vi "Classes Initialization.vi"(7 "LabVIEW Icon in":string, 8 "error in (no error)":errorcluster {"code" min=0 max=0}, 10 "User events":T8, 11 "Ref Cluster":T3) -> (0 "error out":errorcluster {"code" min=0 max=0}, 3 "Data out":T1={"Class"={"Ants"=refnum, "Layer"=refnum, "Templates"=refnum, "Icon"=refnum, "Glyph"=refnum, "Settings"=refnum, "Tools"=refnum}, "Ref"={"Add Layer"=refnum, "Remove Layer"=refnum, "Line Text"=[], "Body Text Spec"=refnum, "DNL_Font"=refnum, "glyph path str"=refnum, "templates path str"=refnum, "Arrow Up"=refnum, "Arrow Down"=refnum, "IE VI Ref"=refnum, "Glyphs tree"=refnum, "Templates tree"=refnum, "Layer Icon Text"=refnum, "Layer Template"=refnum, "Clipboard"=refnum, "BW icon in"=refnum, "Color icon in"=refnum, "Layer Clust"=refnum, "Body Text"=refnum, "DNL_Framework Templates"=refnum, "Search Templates"=refnum, "TextMarker"=refnum, "Tab Control"=refnum, "Search Glyphs"=refnum, "Line Color"=refnum, "DNL_Glyphs []"=refnum, "Fill Color"=refnum, "Tools"=refnum, "Glyphs tree"=refnum, "Icon"=refnum, "Preview"=refnum, "Ants"=refnum, "Terminals"=refnum, "menu reference"=refnum, "LayerNames"=[], "GlyphLoadAnimation"=refnum, "TemplateLoadAnimation"=refnum, "refreshGlyphs"=refnum, "refreshTemplates"=refnum}, "Support"={"AntsRect"={"left"=0, "top"=0, "right"=0, "bottom"=0}, "Mouse Move Coords"={"Horizontal"=0, "Vertical"=0}, "Mouse Down Coords"={"Horizontal"=0, "Vertical"=0}, "Temp Coord"={"Horizontal"=0, "Vertical"=0}, "Action"=enum."Default", "Edge Color"=4914962, "Fill Color"=16860, "Mouse Down?"=FALSE, "Draft Mode?"=FALSE, "Temp Icon"=bytes[3102], "CTRL Pressed"=FALSE, "Move Selection?"=FALSE, "AntsRect Orig"={"left"=0, "top"=0, "right"=0, "bottom"=0}, "Text"="", "TM Set?"=FALSE, "Mouse inside icon?"=FALSE, "Tool (old value)"=0, "Pencil Move Color"=0, "Swap Colors?"=FALSE, "Shift pressed?"=FALSE}})   [LabVIEW 2021]
uses:
  <resource>/plugins/NIIconEditor/Controls/References Cluster.ctl
  <resource>/plugins/NIIconEditor/Controls/IE Data.ctl
  <resource>/plugins/NIIconEditor/Class/Ants/Ants.lvclass
  <resource>/plugins/NIIconEditor/Class/FakedArray/FakedArray.lvclass
  <resource>/plugins/NIIconEditor/Class/Icon Library/Glyph.lvclass
  <resource>/plugins/NIIconEditor/Class/Settings/Settings.lvclass
  <resource>/plugins/NIIconEditor/Class/Tools/Tools Paint.lvclass
  <vilib>/LabVIEW Icon API/lv_icon/Classes/Icon/Icon.lvclass
  <resource>/plugins/NIIconEditor/Controls/IE Classes.ctl
  <resource>/plugins/NIIconEditor/Controls/SupportClass.ctl
  <vilib>/Utility/miscctls.llb/LVPoint32TypeDef.ctl
  <resource>/plugins/NIIconEditor/Controls/SupportClass_Action.ctl
  <vilib>/LabVIEW Icon API/lv_icon/Controls/IEColor.ctl
  <resource>/plugins/NIIconEditor/Controls/ToMoreSpecific_Faked2DArray.ctl
  <resource>/plugins/NIIconEditor/Controls/Undo Redo Action.ctl
  <resource>/plugins/NIIconEditor/Global Variables/Data.vi
panel:
  in  "Data":T1={"Class"={"Ants"=refnum, "Layer"=refnum, "Templates"=refnum, "Icon"=refnum, "Glyph"=refnum, "Settings"=refnum, "Tools"=refnum}, "Ref"={"Add Layer"=refnum, "Remove Layer"=refnum, "Line Text"=[], "Body Text Spec"=refnum, "DNL_Font"=refnum, "glyph path str"=refnum, "templates path str"=refnum, "Arrow Up"=refnum, "Arrow Down"=refnum, "IE VI Ref"=refnum, "Glyphs tree"=refnum, "Templates tree"=refnum, "Layer Icon Text"=refnum, "Layer Template"=refnum, "Clipboard"=refnum, "BW icon in"=refnum, "Color icon in"=refnum, "Layer Clust"=refnum, "Body Text"=refnum, "DNL_Framework Templates"=refnum, "Search Templates"=refnum, "TextMarker"=refnum, "Tab Control"=refnum, "Search Glyphs"=refnum, "Line Color"=refnum, "DNL_Glyphs []"=refnum, "Fill Color"=refnum, "Tools"=refnum, "Glyphs tree"=refnum, "Icon"=refnum, "Preview"=refnum, "Ants"=refnum, "Terminals"=refnum, "menu reference"=refnum, "LayerNames"=[], "GlyphLoadAnimation"=refnum, "TemplateLoadAnimation"=refnum, "refreshGlyphs"=refnum, "refreshTemplates"=refnum}, "Support"={"AntsRect"={"left"=0, "top"=0, "right"=0, "bottom"=0}, "Mouse Move Coords"={"Horizontal"=0, "Vertical"=0}, "Mouse Down Coords"={"Horizontal"=0, "Vertical"=0}, "Temp Coord"={"Horizontal"=0, "Vertical"=0}, "Action"=enum."Default", "Edge Color"=4914962, "Fill Color"=16860, "Mouse Down?"=FALSE, "Draft Mode?"=FALSE, "Temp Icon"=bytes[3102], "CTRL Pressed"=FALSE, "Move Selection?"=FALSE, "AntsRect Orig"={"left"=0, "top"=0, "right"=0, "bottom"=0}, "Text"="", "TM Set?"=FALSE, "Mouse inside icon?"=FALSE, "Tool (old value)"=0, "Pencil Move Color"=0, "Swap Colors?"=FALSE, "Shift pressed?"=FALSE}}
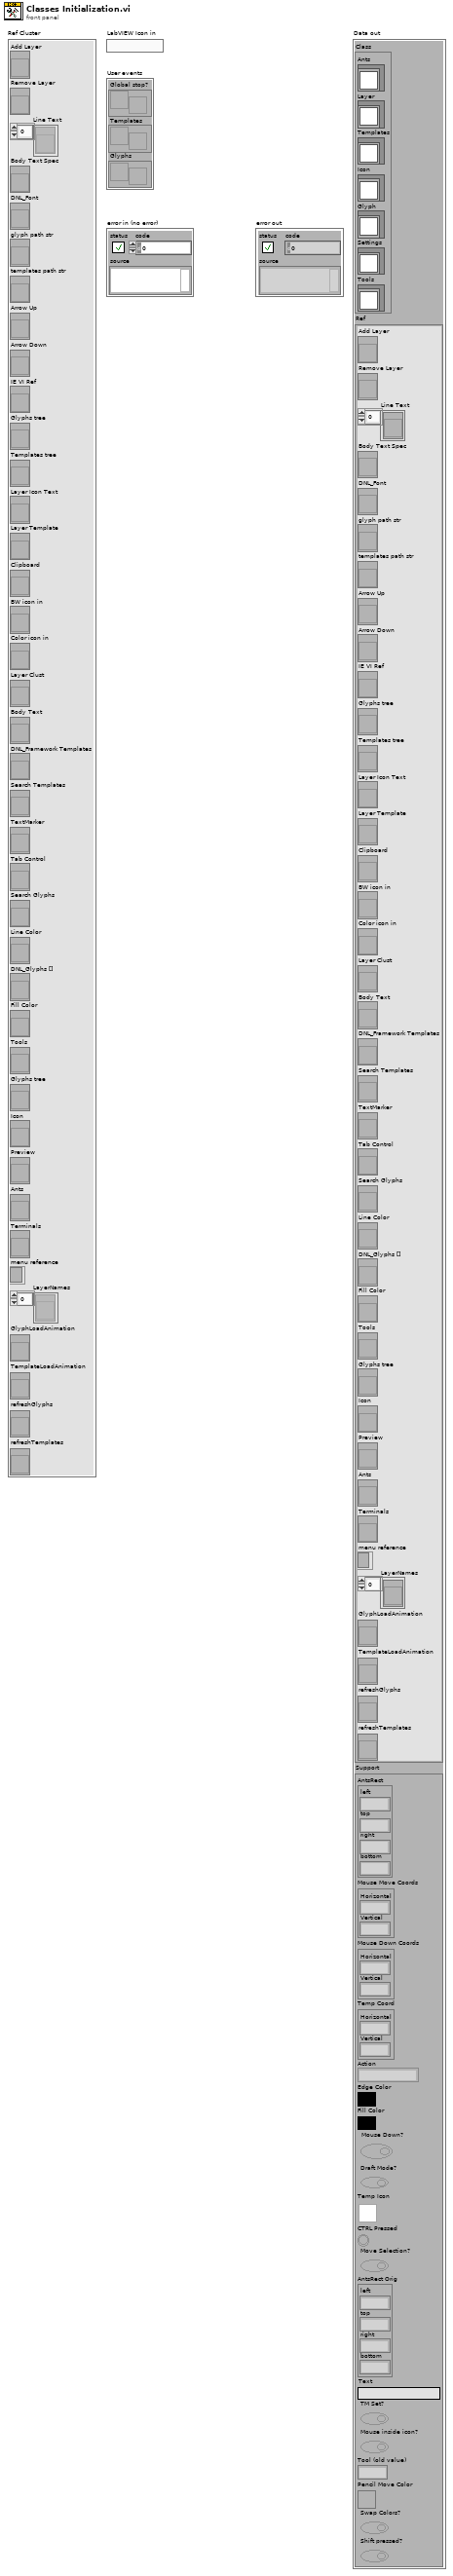
[diagram p1: front panel]
types:
  T1 = typedef "IE Data.ctl" = cluster{"Class":T2, "Ref":T3, "Support":T4}
  T2 = typedef "IE Classes.ctl" = cluster{"Ants":refnum<class "Ants.lvclass">, "Layer":refnum<class "FakedArray.lvclass">, "Templates":refnum<class "FakedArray.lvclass">, "Icon":refnum<class "Icon.lvclass">, "Glyph":refnum<class "Glyph.lvclass">, "Settings":refnum<class "Settings.lvclass">, "Tools":refnum<class "Tools Paint.lvclass">}
  T3 = typedef "References Cluster.ctl" = cluster{"Add Layer":refnum<vi>, "Remove Layer":refnum<vi>, "Line Text":refnum<vi>[], "Body Text Spec":refnum<vi>, "DNL_Font":refnum<vi>, "glyph path str":refnum<vi>, "templates path str":refnum<vi>, "Arrow Up":refnum<vi>, "Arrow Down":refnum<vi>, "IE VI Ref":refnum<vi>, "Glyphs tree":refnum<vi>, "Templates tree":refnum<vi>, "Layer Icon Text":refnum<vi>, "Layer Template":refnum<vi>, "Clipboard":refnum<vi>, "BW icon in":refnum<vi>, "Color icon in":refnum<vi>, "Layer Clust":refnum<vi>, "Body Text":refnum<vi>, "DNL_Framework Templates":refnum<vi>, "Search Templates":refnum<vi>, "TextMarker":refnum<vi>, "Tab Control":refnum<vi>, "Search Glyphs":refnum<vi>, "Line Color":refnum<vi>, "DNL_Glyphs []":refnum<vi>, "Fill Color":refnum<vi>, "Tools":refnum<vi>, "Glyphs tree":refnum<vi>, "Icon":refnum<vi>, "Preview":refnum<vi>, "Ants":refnum<vi>, "Terminals":refnum<vi>, "menu reference":refnum<k9>, "LayerNames":refnum<vi>[], "GlyphLoadAnimation":refnum<vi>, "TemplateLoadAnimation":refnum<vi>, "refreshGlyphs":refnum<vi>, "refreshTemplates":refnum<vi>}
  T4 = typedef "SupportClass.ctl" = cluster{"AntsRect":cluster{"left":i16, "top":i16, "right":i16, "bottom":i16}, "Mouse Move Coords":T5, "Mouse Down Coords":T5, "Temp Coord":T5, "Action":T6, "Edge Color":T7, "Fill Color":T7, "Mouse Down?":bool, "Draft Mode?":bool, "Temp Icon":picture, "CTRL Pressed":bool, "Move Selection?":bool, "AntsRect Orig":cluster{"left":i16, "top":i16, "right":i16, "bottom":i16}, "Text":string, "TM Set?":bool, "Mouse inside icon?":bool, "Tool (old value)":u32, "Pencil Move Color":u32, "Swap Colors?":bool, "Shift pressed?":bool}
  T5 = typedef "LVPoint32TypeDef.ctl" = cluster{"Horizontal":i32, "Vertical":i32}
  T6 = typedef "SupportClass_Action.ctl" = enum16{"Default", "Move Selection", "Glyph Library", "Tool"}
  T7 = typedef "IEColor.ctl" = u32
  T8 = cluster{"Global stop?":refnum<user-event>, "Templates":refnum<user-event>, "Glyphs":refnum<user-event>}
  T9 = typedef "Undo Redo Action.ctl" = enum16{"Init", "Add", "Redo", "Undo", "Undo Preview"}
  T10 = typedef "ToMoreSpecific_Faked2DArray.ctl" = enum16{"Framework Templates", "Layer List"}
  T11 = cluster{"Minimum # of selected elements":u32, "Maximum # of selected elements":u32, "# Rows":u32, "# Cols":u32}
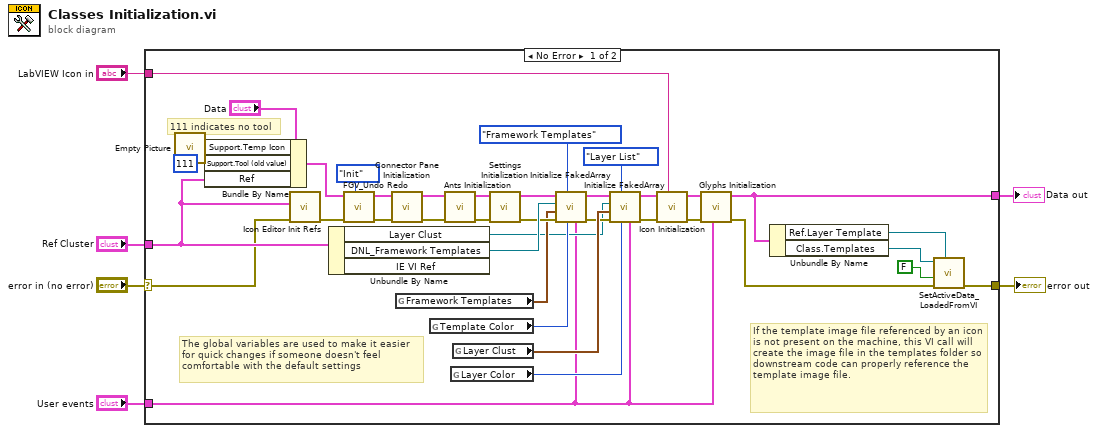
[diagram p0: block diagram]
diagram:
  n1 = case shown="No Error" "error in (no error)" {
    selector: "error in (no error)" -> [w25 w45]
    tunnel: [w11 w45] -> w5
    tunnel: "Ref Cluster" -> [w30 _]
    tunnel: "User events" -> [w32 _]
    tunnel: [w10 _] -> w2
    tunnel: "LabVIEW Icon in" -> [w13 _]
    frame No Error {
      # "If the template image file referenced by an icon is not present on the machine, this VI call will create the image file in the templates folder so downstream code can properly reference the template image file."
      # "The global variables are used to make it easier\nfor quick changes if someone doesn't feel\ncomfortable with the default settings"
      # "111 indicates no tool"
      n2 = call "Empty Picture"() -> ("empty picture"=w21:picture)
      n3 = Bundle By Name(cluster="Data", "Support.Temp Icon"=w21, "Support.Tool (old value)"=u32 111, "Ref"=w30) -> (w14:T1)
      n4 = call <resource>:"Icon Editor Init Refs.vi"("error in (no error)"=w25, "Ref Cluster"=w30) -> ("error out"=w15:errorcluster)  [unwired: 1 in, 8 out]
      n5 = Unbundle By Name(w30) -> ("Layer Clust"=w35:refnum<vi>, "DNL_Framework Templates"=w44:refnum<vi>)  [unwired: 1 out]
      n6 = call <resource>:"FGV_Undo Redo.vi"("Action"=Undo_Redo_Action."Init", "error in (no error)"=w15, "Data in"=w14) -> ("error out"=w16:errorcluster, "Data out"=w17:T1)  [unwired: 1 in, 6 out]
      n7 = call <resource>:"Connector Pane Initialization.vi"("error in (no error)"=w16, "Data in"=w17) -> ("error out"=w33:errorcluster, "Data out"=w26:T1)  [unwired: 8 out]
      n8 = global read "Data.vi" "Framework Templates"() -> (w40:T11)
      n9 = global read "Data.vi" "Template Color"() -> (w39:T7)
      n10 = call <resource>:"Ants Initialization.vi"("error in (no error)"=w33, "Data in"=w26) -> ("error out"=w34:errorcluster, "Data out"=w29:T1)  [unwired: 8 out]
      n11 = global read "Data.vi" "Layer Color"() -> (w37:T7)
      n12 = global read "Data.vi" "Layer Clust"() -> (w38:T11)
      n13 = call <resource>:"Settings Initialization.vi"("error in (no error)"=w34, "Data in"=w29) -> ("error out"=w42:errorcluster, "Data out"=w28:T1)  [unwired: 8 out]
      n14 = call <resource>:"Initialize FakedArray.vi"("User events"=w32, "Color"=w39, "ToMoreSpecific"=ToMoreSpecific_Faked2DArray."Framework Templates", "error in (no error)"=w42, "Data"=w40, "Cluster Refnum"=w44, "Data in"=w28) -> ("error out"=w36:errorcluster, "Data out"=w27:T1)  [unwired: 1 in, 2 out]
      n15 = call <resource>:"Initialize FakedArray.vi"("User events"=w32, "Color"=w37, "ToMoreSpecific"=ToMoreSpecific_Faked2DArray."Layer List", "error in (no error)"=w36, "Data"=w38, "Cluster Refnum"=w35, "Data in"=w27) -> ("error out"=w23:errorcluster, "Data out"=w22:T1)  [unwired: 1 in, 2 out]
      n16 = call <resource>:"Icon Initialization.vi"("LabVIEW Icon in"=w13, "error in (no error)"=w23, "Data in"=w22) -> ("error out"=w20:errorcluster, "Data out"=w19:T1)  [unwired: 7 out]
      n17 = call <resource>:"Glyphs Initialization.vi"("User events"=w32, "error in (no error)"=w20, "Data in"=w19) -> ("error out"=w12:errorcluster, "Data out"=w10:T1)  [unwired: 7 out]
      n18 = Unbundle By Name(w10) -> ("Ref.Layer Template"=w9:refnum<vi>, "Class.Templates"=w8:refnum<class "FakedArray.lvclass">)
      n19 = call <resource>:"SetActiveData_LoadedFromVI.vi"("Layer Template"=w9, "error in (no error)"=w12, "Match?"=FALSE, "FakedArray in"=w8) -> ("error out"=w11:errorcluster)  [unwired: 4 in, 3 out]
    }
    frame Error {
    }
  }
  "error out" <- w5
  "Data out" <- w2
